vi "IsFull.vi"(11 "TypedCircularBuffer in":refnum<class "LogCircularBuffer.lvclass">) -> (2 "Full?":bool, 3 "TypedCircularBuffer out":refnum<class "LogCircularBuffer.lvclass">)   [LabVIEW 2024, in "LogCircularBuffer.lvclass"]
uses:
  LogCircularBuffer.lvclass
  LogCircularBuffer.lvclass/LogCircularBuffer.ctl
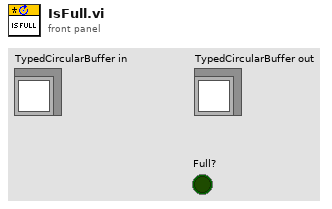
[diagram p1: front panel]
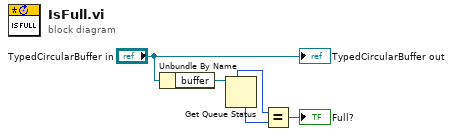
[diagram p0: block diagram]
diagram:
  n1 = Unbundle By Name("TypedCircularBuffer in") -> ("buffer"=w3:refnum<queue>)
  n2 = Get Queue Status(queue=w3) -> (max queue size=w2:i32, # elements in queue=w1:i32)  [unwired: 2 in, 6 out]
  n3 = Equal?(x=w2, y=w1) -> (x = y?=→"Full?":bool)
  "TypedCircularBuffer out" <- "TypedCircularBuffer in"
